vi "pho_DBCheck_LIV_meas_recipe.vi"(0 "V start":dbl=-1.0, 1 "Sweep Direction (Keysight)":i32(ring) items=["Up", "Down"], 5 "V end":dbl=0.4, 7 "points":u16=40, 9 "I compliance sweep":dbl=0.001, 11 "error in (no error)":errorcluster, 12 "sweep delay ms":dbl=500.0) -> (4 "RecipeID":string, 15 "error out":errorcluster)   [LabVIEW 2012]
panel:
  in  "DSN":string="DSN=pho_test"
  out "sql string":string
  # "Sweep Settings"
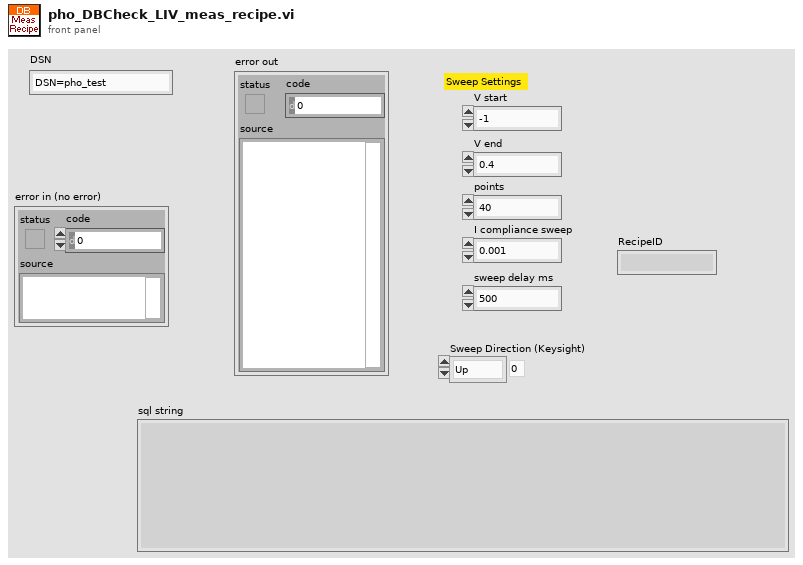
[diagram p1: front panel]
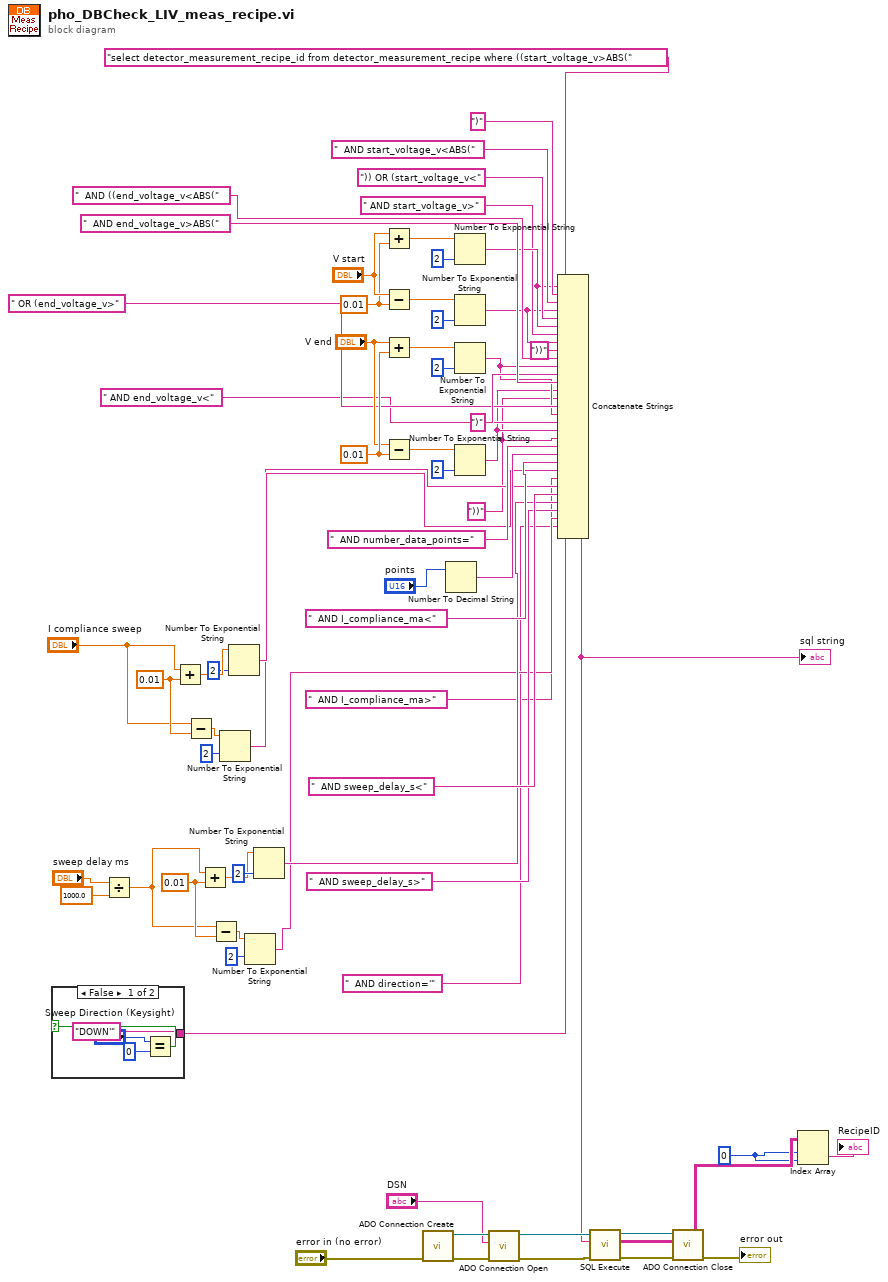
[diagram p0: block diagram]
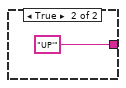
[diagram p2: hidden frame]
diagram:
  w2 = 0 ("index (row)")
  w4 = "))" ("string")
  w31 = 0.01 ("y")
  w43 = 0.01 ("y")
  w49 = 0.01 ("y")
  w60 = 0.01 ("y")
  n1 = Divide(x="sweep delay ms", y=1000.0) -> (x/y=w29:dbl)
  n2 = Equal?(x="Sweep Direction (Keysight)", y=0) -> (x = y?=w19:bool)
  n3 = case shown="False" w19 {
    tunnel: ["DOWN'" ("string") "UP'" ("string")] -> w18
    frame False {
    }
    frame True {
    }
  }
  n4 = Add(x="I compliance sweep", y=w43) -> (x+y=w42:dbl)
  n5 = Subtract(x="I compliance sweep", y=w43) -> (x-y=w40:dbl)
  n6 = Add(x=w29, y=w31) -> (x+y=w32:dbl)
  n7 = Subtract(x=w29, y=w31) -> (x-y=w34:dbl)
  n8 = Number To Exponential String(number=w40, precision (6)=i16 2) -> (E-format string=w27:string)  [unwired: 2 in]
  n9 = Number To Exponential String(number=w42, precision (6)=i16 2) -> (E-format string=w36:string)  [unwired: 2 in]
  n10 = Number To Exponential String(number=w34, precision (6)=i16 2) -> (E-format string=w23:string)  [unwired: 2 in]
  n11 = Number To Exponential String(number=w32, precision (6)=i16 2) -> (E-format string=w25:string)  [unwired: 2 in]
  n12 = Add(x="V start", y=w60) -> (x+y=w58:dbl)
  n13 = Subtract(x="V start", y=w60) -> (x-y=w56:dbl)
  n14 = Add(x="V end", y=w49) -> (x+y=w50:dbl)
  n15 = Subtract(x="V end", y=w49) -> (x-y=w52:dbl)
  n16 = call "ADO Connection Create.vi"("error in (no error)"="error in (no error)") -> ("error out"=w69:errorcluster, "ADODB._Connection Out"=w70:refnum<k7>)  [unwired: 9 in]
  n17 = Number To Decimal String(number="points") -> (decimal integer string=w44:string)  [unwired: 1 in]
  n18 = Number To Exponential String(number=w58, precision (6)=i16 2) -> (E-format string=w12:string)  [unwired: 2 in]
  n19 = Number To Exponential String(number=w56, precision (6)=i16 2) -> (E-format string=w10:string)  [unwired: 2 in]
  n20 = Number To Exponential String(number=w50, precision (6)=i16 2) -> (E-format string=w8:string)  [unwired: 2 in]
  n21 = Number To Exponential String(number=w52, precision (6)=i16 2) -> (E-format string=w6:string)  [unwired: 2 in]
  n22 = call "ADO Connection Open.vi"("error in (no error)"=w69, "ConnectionString"="DSN", "ADODB._Connection In"=w70) -> ("error out"=w67:errorcluster, "ADODB._Connection Out"=w68:refnum<k7>)  [unwired: 7 in]
  n23 = Concatenate Strings("select detector_measurement_recipe_id from detector_measurement_recipe where ((start_voltage_v>ABS(", w12, ")" ("string"), "  AND start_voltage_v<ABS(" ("string"), w10, ")) OR (start_voltage_v<" ("string"), w12, " AND start_voltage_v>" ("string"), w10, "))" ("string"), "  AND ((end_voltage_v<ABS(" ("string"), w8, ")" ("string"), "  AND end_voltage_v>ABS(" ("string"), w6, w4, " OR (end_voltage_v>" ("string"), w8, " AND end_voltage_v<" ("string"), w6, w4, "  AND number_data_points=" ("string"), w44, "  AND I_compliance_ma<" ("string"), w36, "  AND I_compliance_ma>" ("string"), w27, "  AND sweep_delay_s<" ("string"), w25, "  AND sweep_delay_s>" ("string"), w23, "  AND direction='" ("string"), w18) -> (w13:string)
  "sql string" <- w13
  n24 = call "SQL Execute.vi"("error in (no error)"=w67, "Command Text"=w13, "ADODB._Connection In"=w68) -> ("error out"=w65:errorcluster, "Data"=w3:string[][], "ADODB._Connection Out"=w66:refnum<k7>)  [unwired: 5 in, 1 out]
  n25 = call "ADO Connection Close.vi"("error in (no error)"=w65, "ADODB._Connection In"=w66) -> ("error out"=→"error out":errorcluster)  [unwired: 8 in, 1 out]
  n26 = Index Array(array=w3, index (row)=w2, index (col)=w2) -> (element=→"RecipeID":string)
